vi "Do Fold.vi"(9 "Fold Line":string, 10 "Fold Axis":string, 11 "Array in":bool[][](array[boolean])) -> (3 "Array out":bool[][](array[boolean]))   [LabVIEW 2021]
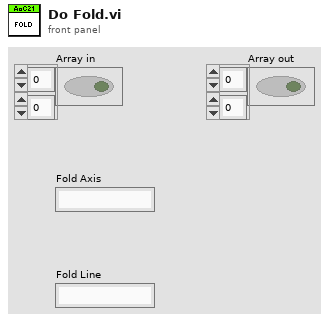
[diagram p1: front panel]
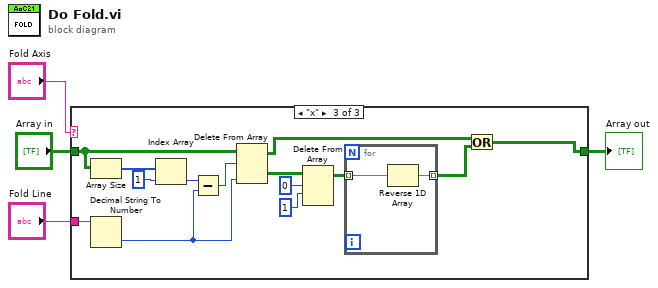
[diagram p0: block diagram]
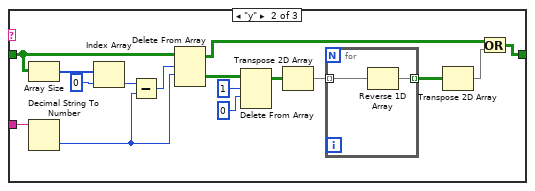
[diagram p3: hidden frame]
diagram:
  n1 = case shown="\"x\"" "Fold Axis" {
    tunnel: "Fold Line" -> [_ w21 w37]
    tunnel: "Array in" -> [w5 w20 w36]
    tunnel: [w5 w6 w25] -> w4
    frame Default {
    }
    frame "y" {
      n2 = Array Size(array=w20) -> (size(s)=w19:i32[])
      n3 = Decimal String To Number(string=w21) -> (number=w12:i32)  [unwired: 2 in, 1 out]
      n4 = Index Array(array=w19, index=0) -> (element=w18:i32)
      n5 = Subtract(x=w18, y=w12) -> (x-y=w15:i32)
      n6 = Delete From Array(array=w20, length=w15, index (row)=w12) -> (deleted portion=w17:bool[][], array with subset deleted=w8:bool[][])  [unwired: 1 in]
      n7 = Delete From Array(array=w17, length=1, index (row)=0 ("disabled index (col)")) -> (array with subset deleted=w11:bool[][])  [unwired: 1 in, 1 out]
      n8 = Transpose 2D Array(2D array=w11) -> (transposed array=w9:bool[][])
      n9 = for {
        tunnel: w9 -> [w23] mode=indexing
        tunnel: [w22] -> w10 mode=indexing
        n10 = Reverse 1D Array(array=w23) -> (reversed array=w22:bool[])
      }
      n11 = Transpose 2D Array(2D array=w10) -> (transposed array=w7:bool[][])
      n12 = Or(x=w8, y=w7) -> (x .or. y?=w6:bool[][])
    }
    frame "x" {
      n13 = Array Size(array=w36) -> (size(s)=w35:i32[])
      n14 = Decimal String To Number(string=w37) -> (number=w24:i32)  [unwired: 2 in, 1 out]
      n15 = Index Array(array=w35, index=1) -> (element=w34:i32)
      n16 = Subtract(x=w34, y=w24) -> (x-y=w31:i32)
      n17 = Delete From Array(array=w36, length=w31, index (col)=w24) -> (deleted portion=w33:bool[][], array with subset deleted=w26:bool[][])  [unwired: 1 in]
      n18 = Delete From Array(array=w33, length=0, index (row)=1 ("disabled index (col)")) -> (array with subset deleted=w28:bool[][])  [unwired: 1 in, 1 out]
      n19 = for {
        tunnel: w28 -> [w39] mode=indexing
        tunnel: [w38] -> w27 mode=indexing
        n20 = Reverse 1D Array(array=w39) -> (reversed array=w38:bool[])
      }
      n21 = Or(x=w26, y=w27) -> (x .or. y?=w25:bool[][])
    }
  }
  "Array out" <- w4
